vi "TS Run Stop.vi"(8 "error in (no error)":errorcluster, 11 "Test Stand in":refnum<class "Generic Test Stand.lvclass">) -> (0 "error out":errorcluster, 3 "Test Stand out":refnum<class "Generic Test Stand.lvclass">)   [LabVIEW 2019, in "Generic Test Stand.lvclass"]
uses:
  Generic Test Stand.lvclass
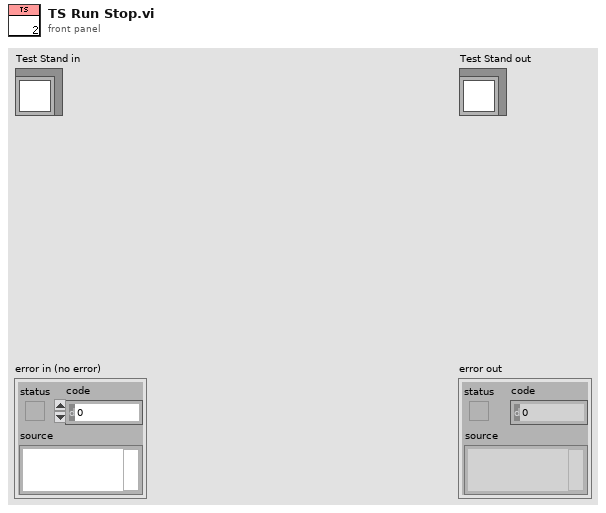
[diagram p1: front panel]
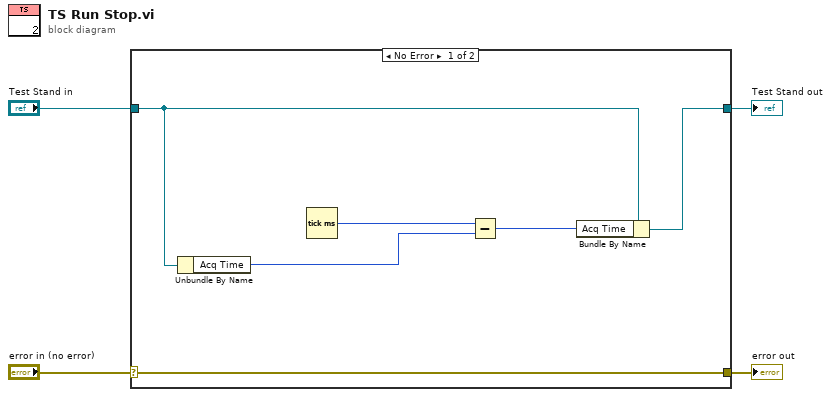
[diagram p0: block diagram]
diagram:
  n1 = case shown="No Error" "error in (no error)" {
    selector: "error in (no error)" -> [w10 w12]
    tunnel: [w10 w12] -> w3
    tunnel: [w9 w11] -> w1
    tunnel: "Test Stand in" -> [w8 w11]
    frame No Error {
      n2 = Unbundle By Name(w8) -> ("Acq Time"=w6:u32)
      n3 = Tick Count (ms)() -> (millisecond timer value=w7:u32)
      n4 = Subtract(x=w7, y=w6) -> (x-y=w5:u32)
      n5 = Bundle By Name(cluster=w8, "Acq Time"=w5) -> (w9:refnum<class "Generic Test Stand.lvclass">)
    }
    frame Error {
    }
  }
  "error out" <- w3
  "Test Stand out" <- w1
